vi "[GV]_STEER0.vi"() -> ()   [LabVIEW 2016]
panel:
  in  "STEER0":u16
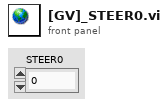
[diagram p1: front panel]
diagram:
